vi "Find Connected Newfis.vi"(6 "error in (no error)":errorcluster) -> (0 "error out":errorcluster, 3 "Connected Board ID's (Newfi)":string[](array[string]))   [LabVIEW 2012]
uses:
  C:/Users/220038920/Desktop/CVS Folder/NI-2010/Trunk/Nufi/Newfi LDN/dll/GeaCommunication.Usb.dll
  Nufi/Newfi LDN/dll/GeaCommunication.Usb.dll
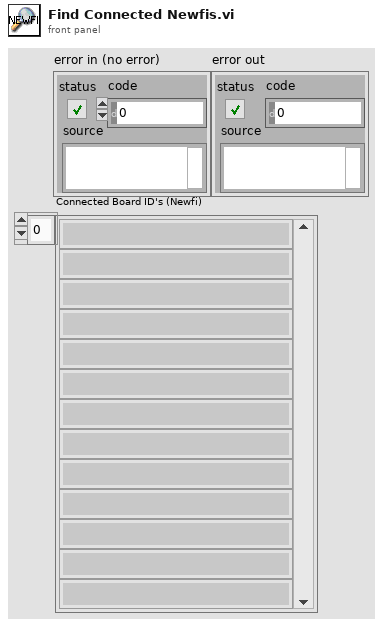
[diagram p1: front panel]
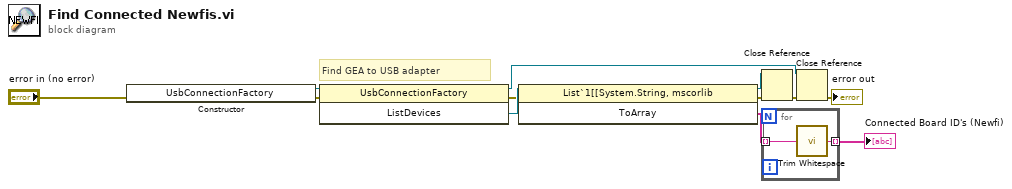
[diagram p0: block diagram]
diagram:
  # "Find GEA to USB adapter"
  n1 = constructor class="UsbConnectionFactory"(error in="error in (no error)") -> (reference out=w11:refnum<k24>, error out=w10:errorcluster)  [unwired: 2 in, 1 out]
  n2 = invoke class="UsbConnectionFactory" method="ListDevices"(reference=w11, error in=w10) -> (reference out=w3:refnum<k24>, error out=w8:errorcluster, "ListDevices"=w12:refnum<k24>)  [unwired: 1 in]
  n3 = invoke class="List`1[[System.String, mscorlib" method="ToArray"(reference=w12, error in=w8) -> (reference out=w5:refnum<k24>, error out=w4:errorcluster, "ToArray"=w7:string[])  [unwired: 1 in]
  n4 = Close Reference(reference=w5, error in (no error)=w4) -> (error out=w2:errorcluster)
  n5 = for {
    tunnel: w7 -> [w14] mode=indexing
    tunnel: [w13] -> w6 mode=indexing
    n6 = call <vilib>:"Trim Whitespace.vi"("string"=w14) -> ("trimmed string"=w13:string)  [unwired: 1 in]
  }
  "Connected Board ID's (Newfi)" <- w6
  n7 = Close Reference(reference=w3, error in (no error)=w2) -> (error out=→"error out":errorcluster)
